vi "black box state code.vi"(10 "value in":dbl, 11 "state control in":T1) -> (2 "value out":dbl, 3 "state control out":T1)   [LabVIEW 2013, in "user tag bus module.lvclass"]
uses:
  user tag bus module.lvclass
  state control.ctl
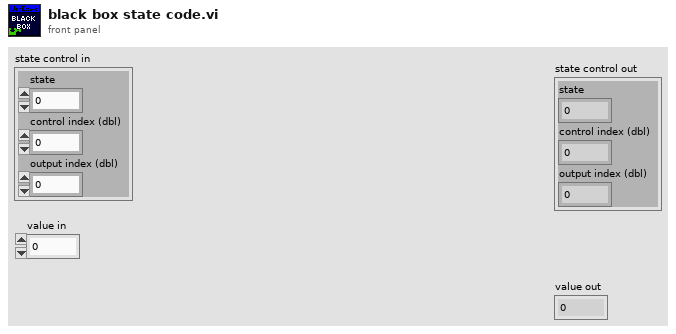
[diagram p1: front panel]
types:
  T1 = typedef "user tag bus module.lvclass/state control.ctl" = cluster{"state":u8, "control index (dbl)":i32, "output index (dbl)":i32}
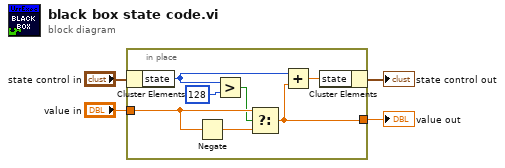
[diagram p0: block diagram]
diagram:
  n1 = in-place {
    in-place-border: [w11] -> w4
    in-place-border: "value in" -> [w9]
    n2 = in-place-cluster #1("state control in") -> ("state"=w6:u8)
    n3 = Negate(x=w9) -> (-x=w10:dbl)
    n4 = Greater?(x=w6, y=u8 128) -> (0:w8:bool)
    n5 = Select(t=w9, s=w8, f=w10) -> (s? t:f=w11:dbl)
    n6 = Add(x=w6, y=w11) -> (x+y=w5:dbl)
    n7 = in-place-cluster #1("state"=w5) -> (→"state control out":T1)
  }
  "value out" <- w4
